vi "Acquisition Message Loop.vi"(8 "error in (no error)":errorcluster, 9 "queue out":refnum<queue>, 10 "Data Notifier":refnum<notifier>, 11 "Message Queues":T1) -> (0 "error out":errorcluster)   [LabVIEW 2018, in "Acquisition.lvlib"]
doc: "Message loop for handling messages pertaining to the acquisition of data from the hardware."
uses:
  Acquisition.lvlib
  support/Message Queue/Message Cluster.ctl
  Acquisition State.ctl
  GlobalVariable/GlobalDisconnected.vi
  GlobalVariable/GlobalPowerByTime.vi
  GlobalVariable/GlobalPosXbyTime.vi
  GlobalVariable/GlobalPosYbyTime.vi
  GlobalVariable/GlobalProfileByTime.vi
  GlobalVariable/GlobalTensionByTime.vi
  GlobalVariable/GlobalTemperatureByTime.vi
  GlobalVariable/Globalt0.vi
  support/Message Queue/Enqueue Message (Single).vi
  GlobalVariable/GlobalLongueurOnde.vi
  GlobalVariable/GlobalTimeStep.vi
  <vilib>/Utility/error.llb/Error Cluster From Error Code.vi
  <vilib>/ErrorRing/Error Ring.xnode
  support/Message Queue/Message Queue.lvlib
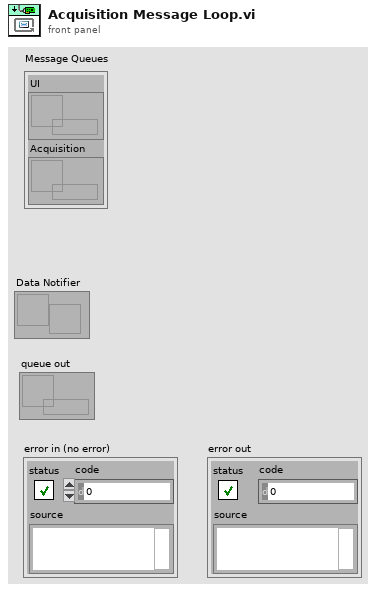
[diagram p1: front panel]
types:
  T1 = cluster{"UI":refnum<queue>, "Acquisition":refnum<queue>}
  T2 = typedef "Acquisition.lvlib/Acquisition State.ctl" = enum16{"Idle", "Acquiring"}
  T3 = enum16{"open", "replace", "create", "open or create", "replace or create", "replace or create with confirmation"}
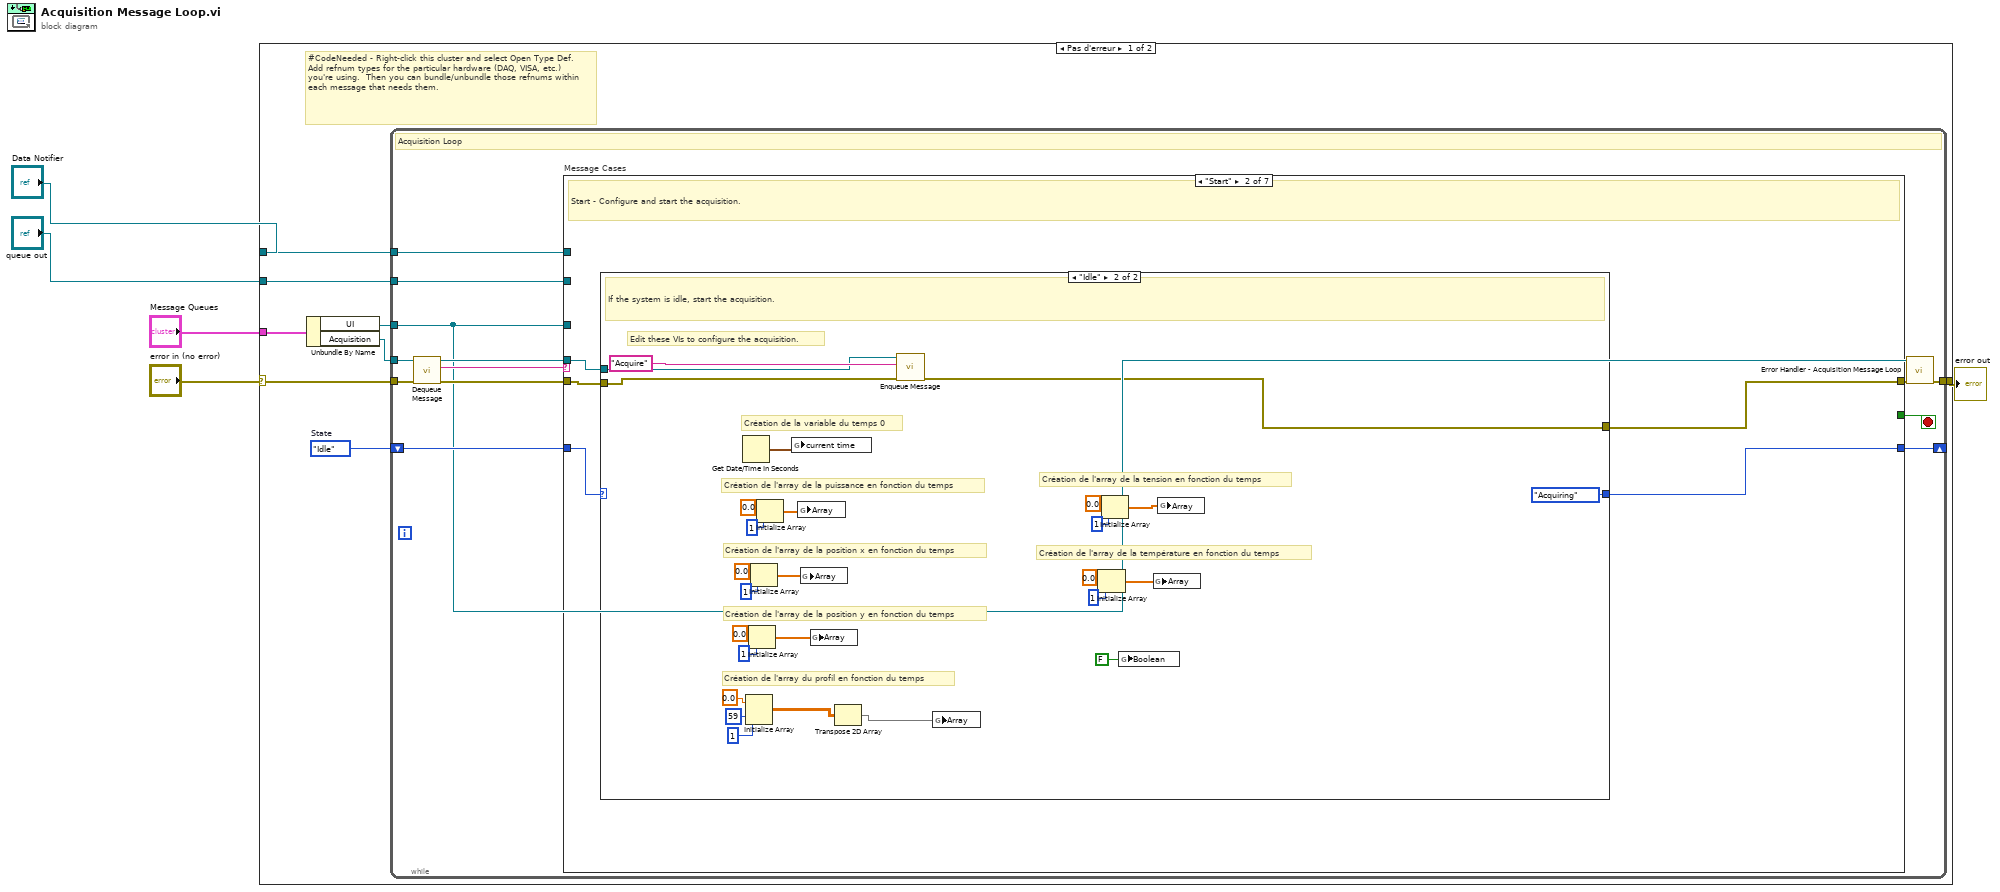
[diagram p0: block diagram]
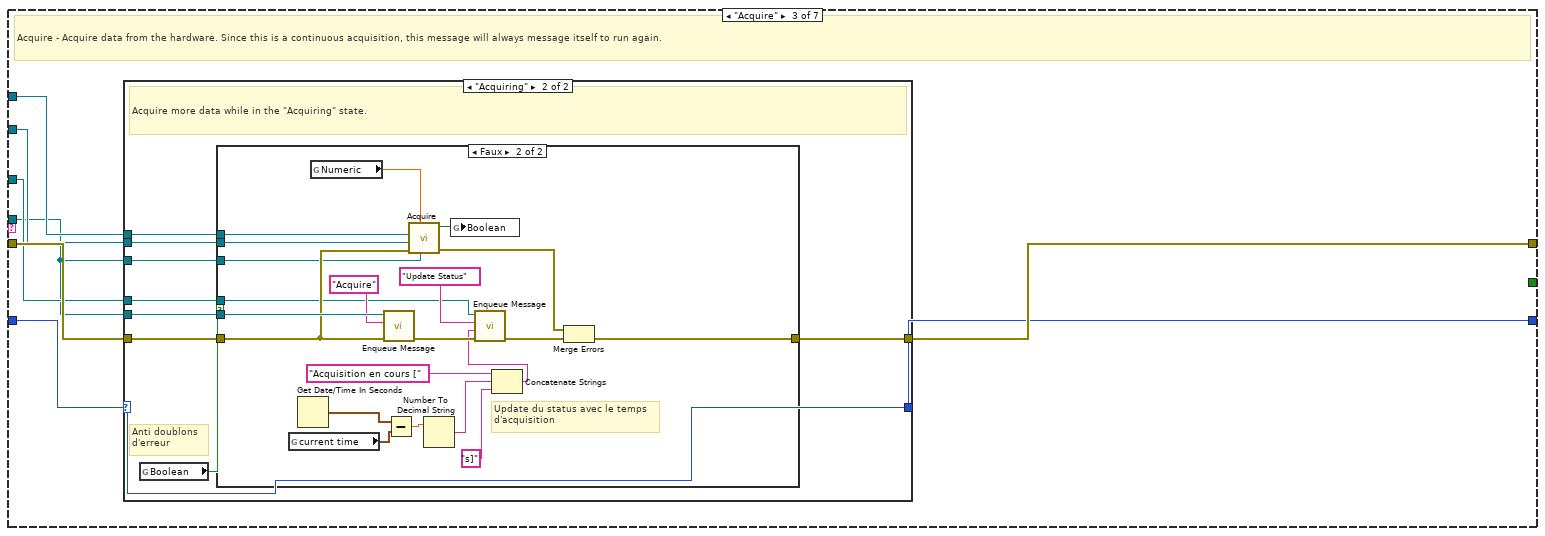
[diagram p4: hidden frame]
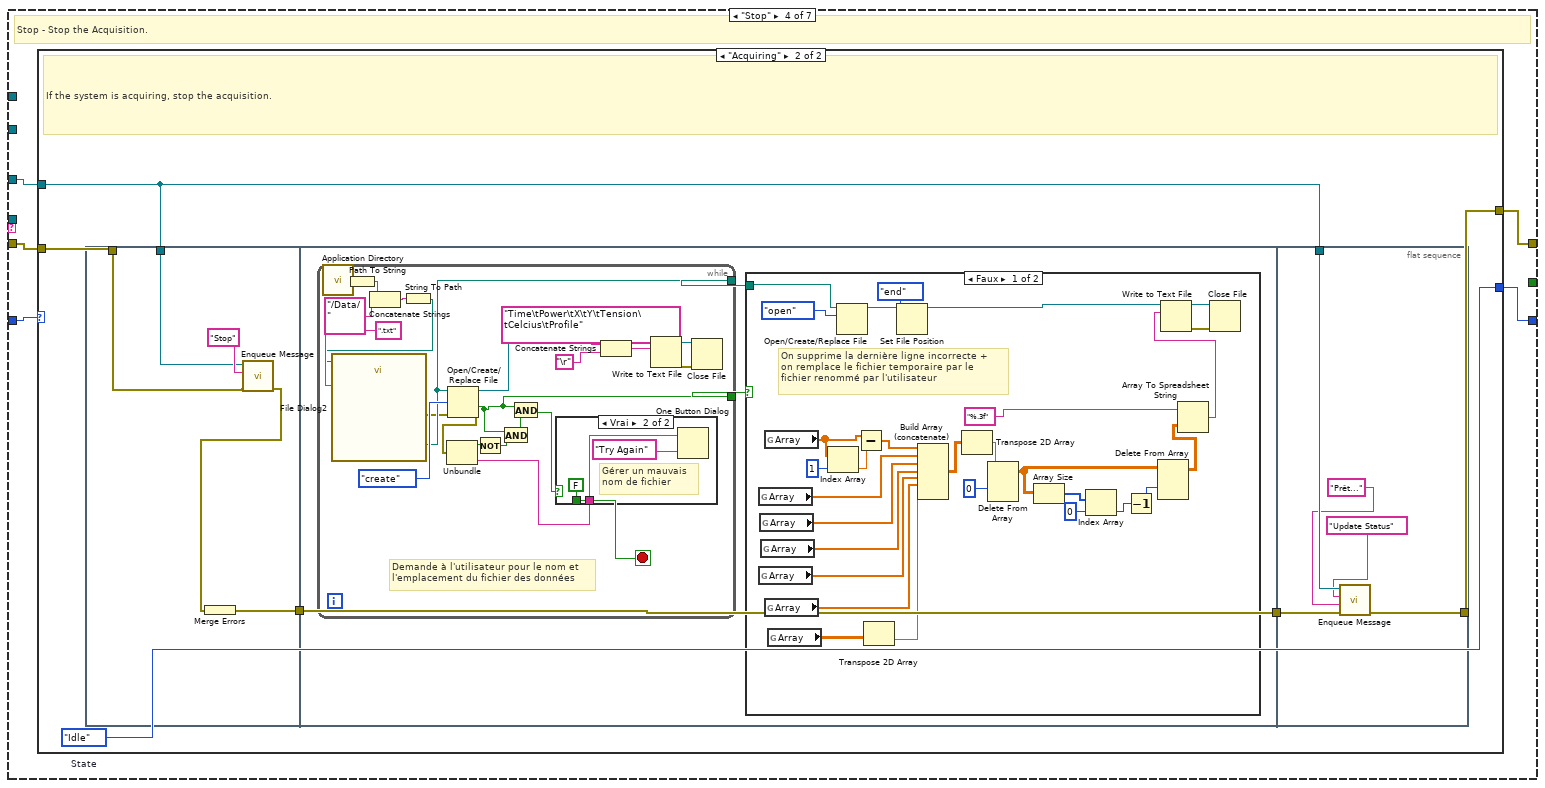
[diagram p7: hidden frame]
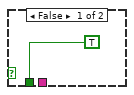
[diagram p10: hidden frame]
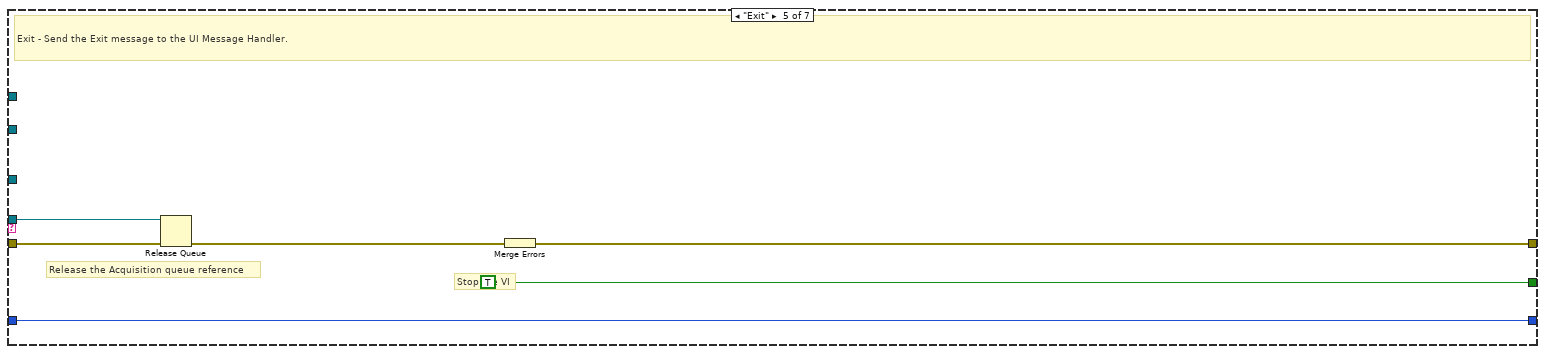
[diagram p11: hidden frame]
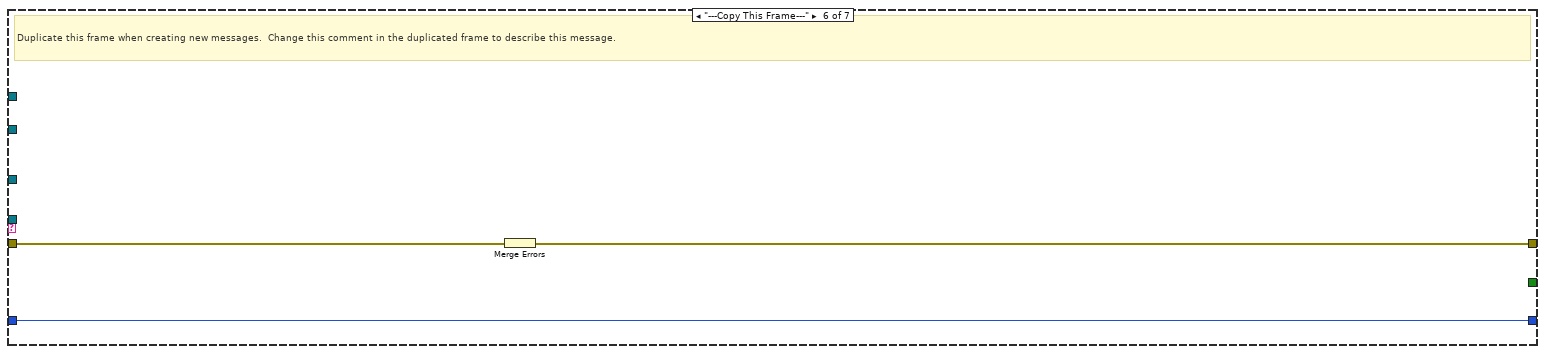
[diagram p12: hidden frame]
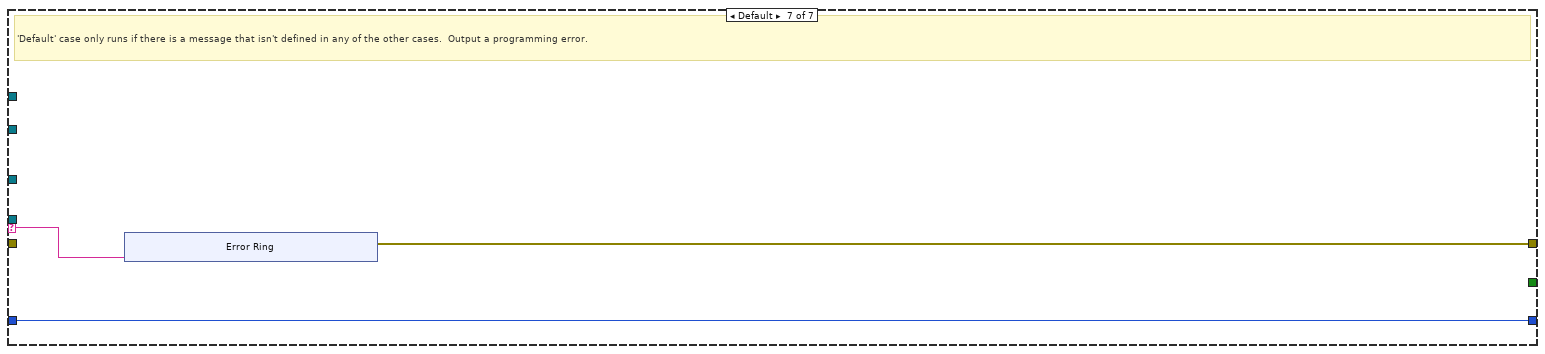
[diagram p13: hidden frame]
diagram:
  n1 = case shown="Pas d'erreur" "error in (no error)" {
    selector: "error in (no error)" -> [w10 w205]
    tunnel: "Message Queues" -> [w13 _]
    tunnel: [w11 w205] -> w4
    tunnel: "Data Notifier" -> [w8 _]
    tunnel: "queue out" -> [w7 _]
    frame No Error {
      w6 = Acquisition_State."Idle"  # State
      # "#CodeNeeded - Right-click this cluster and select Open Type Def.  Add refnum types for the particular hardware (DAQ, VISA, etc.) you're using.  Then you can bundle/unbundle those refnums within each message that needs them."
      n2 = Unbundle By Name(w13) -> ("UI"=w9:refnum<queue>, "Acquisition"=w12:refnum<queue>)
      n3 = while {
        tunnel: w12 -> [w14]
        tunnel: w9 -> [w15]
        tunnel: w8 -> [w22]
        tunnel: w7 -> [w21]
        shift-right: [w19] -> _
        shift-left: w6 -> [w20]
        tunnel: w10 -> [w25]
        tunnel: [w18] -> w11
        stop <- w26 stop-if-true
        # "Acquisition Loop"
        n4 = call "Dequeue Message.vi"("error in (no error)"=w25, "Message Queue"=w14) -> ("error out"=w24:errorcluster, "Message"=w23:string, "dup Message Queue"=w16:refnum<queue>)  [unwired: 6 in, 1 out]
        n5 = case "Message Cases" shown="\"Start\"" w23 {
          selector: w23 -> [_ _ _ _ _ _ w195]
          tunnel: w16 -> [_ w31 w63 _ w187 _ _]
          tunnel: w24 -> [w28 w32 w69 w107 w189 w194 _]
          tunnel: [w28 w33 w70 w105 w190 w193 w196] -> w17
          tunnel: [_ _ _ _ TRUE _ _] -> w26
          tunnel: w15 -> [_ _ w64 w106 _ _ _]
          tunnel: w22 -> [_ _ w68 _ _ _ _]
          tunnel: w21 -> [_ _ w67 _ _ _ _]
          tunnel: w20 -> [w27 w29 w65 w108 w186 w192 w197]
          tunnel: [w27 w30 w66 w104 w186 w192 w197] -> w19
          frame "Initialize" {
            # "Initialize  - Initialize is currently a no-op.  The hardware initialization takes place in the 'Start' message."
          }
          frame "Start" {
            # "Start - Configure and start the acquisition."
            n6 = case shown="\"Idle\"" w29 {
              selector: w29 -> [w34 _]
              tunnel: [w35 w58] -> w33
              tunnel: w32 -> [w35 w62]
              tunnel: w31 -> [_ w59]
              tunnel: [w34 Acquisition_State."Acquiring" ("Acquisition State")] -> w30
              frame "Acquiring" {
                # "The system is already acquiring. Ignore the \"Start\" message."
              }
              frame "Idle" {
                # "Création de l'array de la température en fonction du temps"
                # "Création de l'array de la tension en fonction du temps"
                # "Création de la variable du temps 0"
                # "Création de l'array du profil en fonction du temps"
                # "Création de l'array de la position y en fonction du temps"
                # "Création de l'array de la position x en fonction du temps"
                # "Création de l'array de la puissance en fonction du temps"
                # "Edit these VIs to configure the acquisition."
                # "If the system is idle, start the acquisition."
                n7 = Get Date/Time In Seconds() -> (seconds since 1Jan1904=w42:timestamp)
                n8 = Initialize Array(0.0, 59 ("dimension size"), 1 ("dimension size")) -> (w54:dbl[][])
                n9 = Initialize Array(0.0, 1) -> (w55:dbl[])
                n10 = Initialize Array(0.0, 1) -> (w56:dbl[])
                n11 = Initialize Array(0.0, 1) -> (w57:dbl[])
                n12 = global write "Globalt0.vi" "current time"(w42) -> ()
                n13 = global write "GlobalPowerByTime.vi" "Array"(w57) -> ()
                n14 = global write "GlobalPosXbyTime.vi" "Array"(w56) -> ()
                n15 = global write "GlobalPosYbyTime.vi" "Array"(w55) -> ()
                n16 = Transpose 2D Array(2D array=w54) -> (transposed array=w53:dbl[][])
                n17 = call-poly "Enqueue Message.vi"("error in (no error)"=w62, "Message"="Acquire", "Message Queue"=w59) -> ("error out"=w58:errorcluster)  [unwired: 7 in, 1 out]
                n18 = global write "GlobalProfileByTime.vi" "Array"(w53) -> ()
                n19 = Initialize Array(0.0, 1) -> (w36:dbl[])
                n20 = Initialize Array(0.0, 1) -> (w37:dbl[])
                n21 = global write "GlobalDisconnected.vi" "Boolean"(FALSE) -> ()
                n22 = global write "GlobalTemperatureByTime.vi" "Array"(w36) -> ()
                n23 = global write "GlobalTensionByTime.vi" "Array"(w37) -> ()
              }
            }
          }
          frame "Acquire" {
            # "Acquire - Acquire data from the hardware. Since this is a continuous acquisition, this message will always message itself to run again."
            n24 = case shown="\"Acquiring\"" w65 {
              selector: w65 -> [w71 w77]
              tunnel: [w72 w81] -> w70
              tunnel: w63 -> [_ w80]
              tunnel: w69 -> [w72 w76]
              tunnel: w68 -> [_ w79]
              tunnel: w67 -> [_ w78]
              tunnel: [w71 w77] -> w66
              tunnel: w64 -> [_ w75]
              tunnel: w63 -> [_ w74]
              frame "Idle" {
                # "Ignore \"Acquire\" messages when the acquisition is idle."
              }
              frame "Acquiring" {
                # "Anti doublons\nd'erreur"
                # "Acquire more data while in the \"Acquiring\" state."
                n25 = global read "GlobalDisconnected.vi" "Boolean"() -> (w73:bool)
                n26 = case shown="Faux" w73 {
                  tunnel: [w82 w103] -> w81
                  tunnel: w80 -> [_ w102]
                  tunnel: w79 -> [_ w99]
                  tunnel: w78 -> [_ w98]
                  tunnel: w76 -> [w82 w97]
                  tunnel: w75 -> [_ w86]
                  tunnel: w74 -> [_ w85]
                  frame True {
                  }
                  frame False {
                    # "Update du status avec le temps\nd'acquisition"
                    n27 = global read "Globalt0.vi" "current time"() -> (w92:timestamp)
                    n28 = Get Date/Time In Seconds() -> (seconds since 1Jan1904=w91:timestamp)
                    n29 = global read "GlobalLongueurOnde.vi" "Numeric"() -> (w84:dbl)
                    n30 = call-poly "Enqueue Message.vi"("error in (no error)"=w97, "Message"="Acquire", "Message Queue"=w102) -> ("error out"=w95:errorcluster)  [unwired: 7 in, 1 out]
                    n31 = Subtract(x=w91, y=w92) -> (x-y=w93:dbl)
                    n32 = call "Acquire.vi"("Acquisition"=w85, "Longueur d'onde"=w84, "error in (no error)"=w97, "Data Queue"=w98, "Data Notifier"=w99) -> ("error out"=w101:errorcluster, "Disconnected"=w83:bool)  [unwired: 5 in]
                    n33 = Number To Decimal String(number=w93) -> (decimal integer string=w90:string)  [unwired: 1 in]
                    n34 = global write "GlobalDisconnected.vi" "Boolean"(w83) -> ()
                    n35 = Concatenate Strings("Acquisition en cours [", w90, "s]" ("string")) -> (w88:string)
                    n36 = call-poly "Enqueue Message.vi"("error in (no error)"=w95, "Message Data"=w88, "Message"="Update Status", "Message Queue"=w86) -> ("error out"=w96:errorcluster)  [unwired: 6 in, 1 out]
                    n37 = Merge Errors(w101, w96) -> (w103:errorcluster)
                  }
                }
              }
            }
          }
          frame "Stop" {
            # "Stop - Stop the Acquisition."
            n38 = case shown="\"Acquiring\"" w108 {
              selector: w108 -> [w110 _]
              tunnel: w107 -> [w109 w115]
              tunnel: w106 -> [_ w111]
              tunnel: [w109 w114] -> w105
              tunnel: [w110 w113] -> w104
              frame "Idle" {
                # "The system is already idle. Ignore the \"Stop\" message."
              }
              frame "Acquiring" {
                w113 = Acquisition_State."Idle"  # State
                # "If the system is acquiring, stop the acquisition."
                n39 = flat-sequence {
                  tunnel: [w121] -> w116
                  tunnel: w111 -> [w118]
                  tunnel: w115 -> [w117]
                  tunnel: w116 -> [w123]
                  tunnel: [w123] -> w112
                  tunnel: [w184] -> w114
                  tunnel: w112 -> [w185]
                  tunnel: w111 -> [w183]
                  frame #0 {
                    n40 = call-poly "Enqueue Message.vi"("error in (no error)"=w117, "Message"="Stop", "Message Queue"=w118) -> ("error out"=w120:errorcluster)  [unwired: 7 in, 1 out]
                    n41 = Merge Errors(w120) -> (w121:errorcluster)
                  }
                  frame #1 {
                    n42 = while {
                      tunnel: [w171] -> w124
                      tunnel: [w161] -> w122
                      stop <- w167 stop-if-true
                      # "Demande à l'utilisateur pour le nom et\nl'emplacement du fichier des données"
                      n43 = call <vilib>:"Application Directory.vi"() -> ("Application Directory"=w174:path)
                      n44 = Path To String(path=w174) -> (string=w175:string)
                      n45 = Concatenate Strings(w175, "/Data/") -> (w176:string)
                      n46 = String To Path(string=w176) -> (path=w160:path)
                      n47 = call "File Dialog2"("start path"=w160, "pattern (all files)"=".txt") -> ("selected path"=w171:path, "error out"=w169:errorcluster)  [unwired: 10 in, 2 out]
                      n48 = Open/Create/Replace File(file path (use dialog)=w171, error in=w169, operation (0:open)=T3."create") -> (refnum out=w156:refnum<file>, cancelled=w161:bool, error out=w166:errorcluster)  [unwired: 3 in]
                      n49 = Unbundle(w166) -> ("status"=w165:bool, "source"=w168:string)  [unwired: 1 out]
                      n50 = Not(x=w165) -> (.not. x?=w164:bool)
                      n51 = And(x=w161, y=w164) -> (x .and. y?=w163:bool)
                      n52 = And(x=w161, y=w163) -> (x .and. y?=w162:bool)
                      n53 = case shown="Vrai" w162 {
                        tunnel: w168 -> [_ w180]
                        tunnel: [TRUE FALSE] -> w167
                        frame False {
                        }
                        frame True {
                          # "Gérer un mauvais \nnom de fichier"
                          n54 = One Button Dialog(message=w180, button name ("OK")="Try Again") -> ()  [unwired: 1 out]
                        }
                      }
                      n55 = Concatenate Strings("Time\tPower\tX\tY\tTension\tCelcius\tProfile", "\r") -> (w159:string)
                      n56 = Write to Text File(file (use dialog)=w156, text=w159) -> (refnum out=w155:refnum<file>, error out=w154:errorcluster)  [unwired: 2 in, 1 out]
                      n57 = Close File(refnum=w155, error in=w154) -> ()  [unwired: 2 out]
                    }
                    n58 = case shown="Faux" w122 {
                      tunnel: w124 -> [w147 _]
                      frame False {
                        # "On supprime la dernière ligne incorrecte + \non remplace le fichier temporaire par le \nfichier renommé par l'utilisateur"
                        n59 = global read "GlobalPowerByTime.vi" "Array"() -> (w146:dbl[])
                        n60 = global read "GlobalTensionByTime.vi" "Array"() -> (w126:dbl[])
                        n61 = global read "GlobalPosXbyTime.vi" "Array"() -> (w145:dbl[])
                        n62 = global read "GlobalPosYbyTime.vi" "Array"() -> (w144:dbl[])
                        n63 = global read "GlobalTimeStep.vi" "Array"() -> (w134:dbl[])
                        n64 = global read "GlobalTemperatureByTime.vi" "Array"() -> (w125:dbl[])
                        n65 = global read "GlobalProfileByTime.vi" "Array"() -> (w142:dbl[][])
                        n66 = Index Array(array=w134, index=1) -> (element=w135:dbl)
                        n67 = Open/Create/Replace File(file path (use dialog)=w147, operation (0:open)=T3."open") -> (refnum out=w151:refnum<file>)  [unwired: 4 in, 2 out]
                        n68 = Subtract(x=w134, y=w135) -> (x-y=w133:dbl[])
                        n69 = Transpose 2D Array(2D array=w142) -> (transposed array=w141:dbl[][])
                        n70 = Set File Position(refnum=w151, from (0:start)=enum16{"start", "end", "current"}."end") -> (refnum out=w153:refnum<file>)  [unwired: 2 in, 1 out]
                        n71 = Build Array (concatenate)(w133, w146, w145, w144, w126, w125, w141) -> (w143:dbl[][])
                        n72 = Transpose 2D Array(2D array=w143) -> (transposed array=w137:dbl[][])
                        n73 = Delete From Array(array=w137, index (row)=0) -> (array with subset deleted=w128:dbl[][])  [unwired: 2 in, 1 out]
                        n74 = Array Size(array=w128) -> (size(s)=w132:i32[])
                        n75 = Index Array(array=w132, index=0) -> (element=w130:i32)
                        n76 = Decrement(x=w130) -> (x-1=w129:i32)
                        n77 = Delete From Array(array=w128, index (row)=w129) -> (array with subset deleted=w127:dbl[][])  [unwired: 2 in, 1 out]
                        n78 = Array To Spreadsheet String(array=w127, 3:"%.3f" ("format string")) -> (spreadsheet string=w152:string)  [unwired: 1 in]
                        n79 = Write to Text File(file (use dialog)=w153, text=w152) -> (refnum out=w140:refnum<file>, error out=w139:errorcluster)  [unwired: 2 in, 1 out]
                        n80 = Close File(refnum=w140, error in=w139) -> ()  [unwired: 2 out]
                      }
                      frame True {
                      }
                    }
                  }
                  frame #2 {
                    n81 = call-poly "Enqueue Message.vi"("error in (no error)"=w185, "Message Data"="Prêt...", "Message"="Update Status", "Message Queue"=w183) -> ("error out"=w184:errorcluster)  [unwired: 6 in, 1 out]
                  }
                }
              }
            }
          }
          frame "Exit" {
            # "Release the Acquisition queue reference"
            # "Stop the VI"
            # "Exit - Send the Exit message to the UI Message Handler."
            n82 = Release Queue(queue=w187, error in (no error)=w189) -> (error out=w188:errorcluster)  [unwired: 1 in, 2 out]
            n83 = Merge Errors(w188) -> (w190:errorcluster)
          }
          frame "---Copy This Frame---" {
            # "Duplicate this frame when creating new messages.  Change this comment in the duplicated frame to describe this message."
            n84 = Merge Errors(w194) -> (w193:errorcluster)
          }
          frame Default {
            # "'Default' case only runs if there is a message that isn't defined in any of the other cases.  Output a programming error."
            n85 = xnode "Error Ring"("paramètre 0"=w195) -> ("sortie d'erreur"=w196:errorcluster)
          }
        }
        n86 = call "Error Handler - Acquisition Message Loop.vi"("error in (no error)"=w17, "Message Queue"=w15) -> ("dup error in"=w18:errorcluster)  [unwired: 8 in, 1 out]
      }
    }
    frame Error {
    }
  }
  "error out" <- w4
